vi "Configure Scalar Mixer Calibration.vi"(6 "Method (0: 1-port Calibration)":u16(ring) items=["1-port Calibration", "2-port Calibration"], 7 "Channel (1)":i32=1, 8 "error in (no error)":errorcluster, 9 "Port 2 (1)":i32=1, 10 "Port 1 (1)":i32=1, 11 "VISA resource name":refnum<visa-resource-name>) -> (0 "error out":errorcluster, 3 "VISA resource name out":refnum<visa-resource-name>)   [LabVIEW 2018, in "Agilent ENA Series.lvlib"]
doc: "Configures the scalar-mixer calibration.\n\n<b>Note:</b>\nThis VI is not supported by the E5063A and E5080A."
uses:
  Agilent ENA Series.lvlib
panel:
  # "Note:\nThis VI is not supported by the E5063A and E5080A."
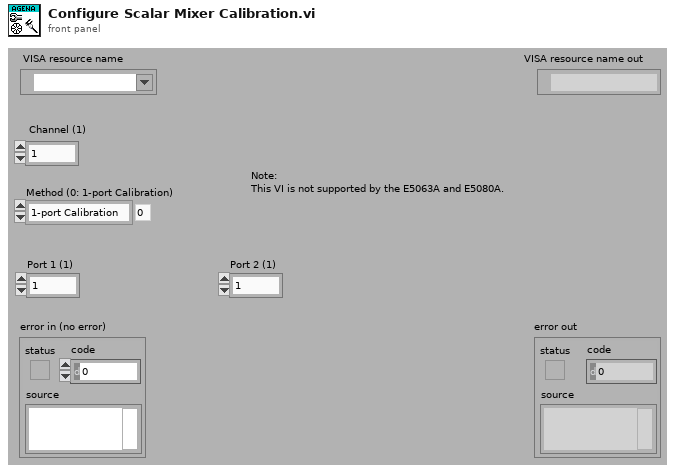
[diagram p1: front panel]
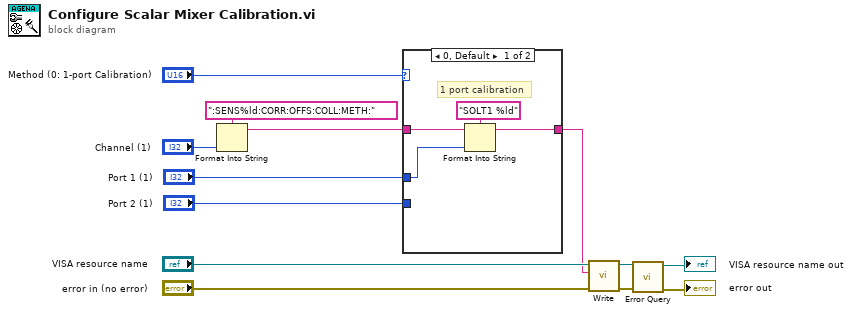
[diagram p0: block diagram]
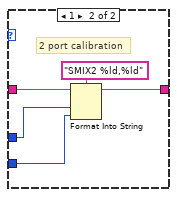
[diagram p2: hidden frame]
diagram:
  n1 = Format Into String(format string=":SENS%ld:CORR:OFFS:COLL:METH:", "Channel (1)") -> (resulting string=w9:string)  [unwired: 2 in, 1 out]
  n2 = case shown="0, Default" "Method (0: 1-port Calibration)" {
    tunnel: w9 -> [w16 w21]
    tunnel: "Port 1 (1)" -> [w15 w20]
    tunnel: "Port 2 (1)" -> [_ w18]
    tunnel: [w14 w19] -> w6
    frame 0, Default {
      # "1 port calibration"
      n3 = Format Into String(format string="SOLT1 %ld", initial string=w16, w15) -> (resulting string=w14:string)  [unwired: 1 in, 1 out]
    }
    frame 1 {
      # "2 port calibration"
      n4 = Format Into String(format string="SMIX2 %ld,%ld", initial string=w21, w20, w18) -> (resulting string=w19:string)  [unwired: 1 in, 1 out]
    }
  }
  n5 = call "Write.vi"("error in (no error)"="error in (no error)", "String ()"=w6, "VISA resource name"="VISA resource name") -> ("error out"=w3:errorcluster, "VISA resource name out"=w4:refnum<visa-resource-name>)  [unwired: 6 in, 1 out]
  n6 = call "Error Query.vi"("error in (no error)"=w3, "VISA resource name"=w4) -> ("error out"=→"error out":errorcluster, "VISA resource name out"=→"VISA resource name out":refnum<visa-resource-name>)  [unwired: 6 in, 2 out]
